vi "Demo.vi"() -> ()   [LabVIEW 2021]
uses:
  Z:/Samples/Examples/WindowsDesktop/bin/Debug/UnderAutomation.UniversalRobots.dll
  WindowsDesktop/bin/Debug/UnderAutomation.UniversalRobots.dll
panel:
  in  "Connect 2":bool
  in  "Program to load":string
  in  "Power on 6":bool
  in  "Power on 5":bool
  in  "Power on 4":bool
  in  "Power on 3":bool
  in  "Power on 2":bool
  in  "Send script":bool
  in  "Script":string
  in  "Connect":bool
  in  "IP":string
  in  "Power on":bool
  out "Z":dbl
  out "Y":dbl
  out "X":dbl
  # "Robot TCP position :"
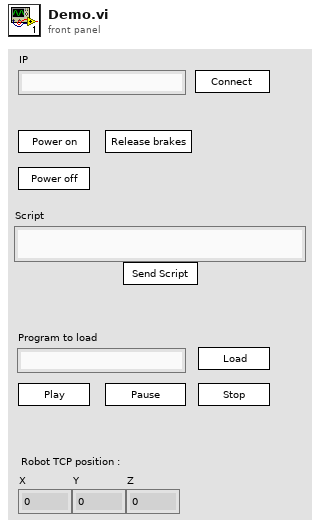
[diagram p1: front panel]
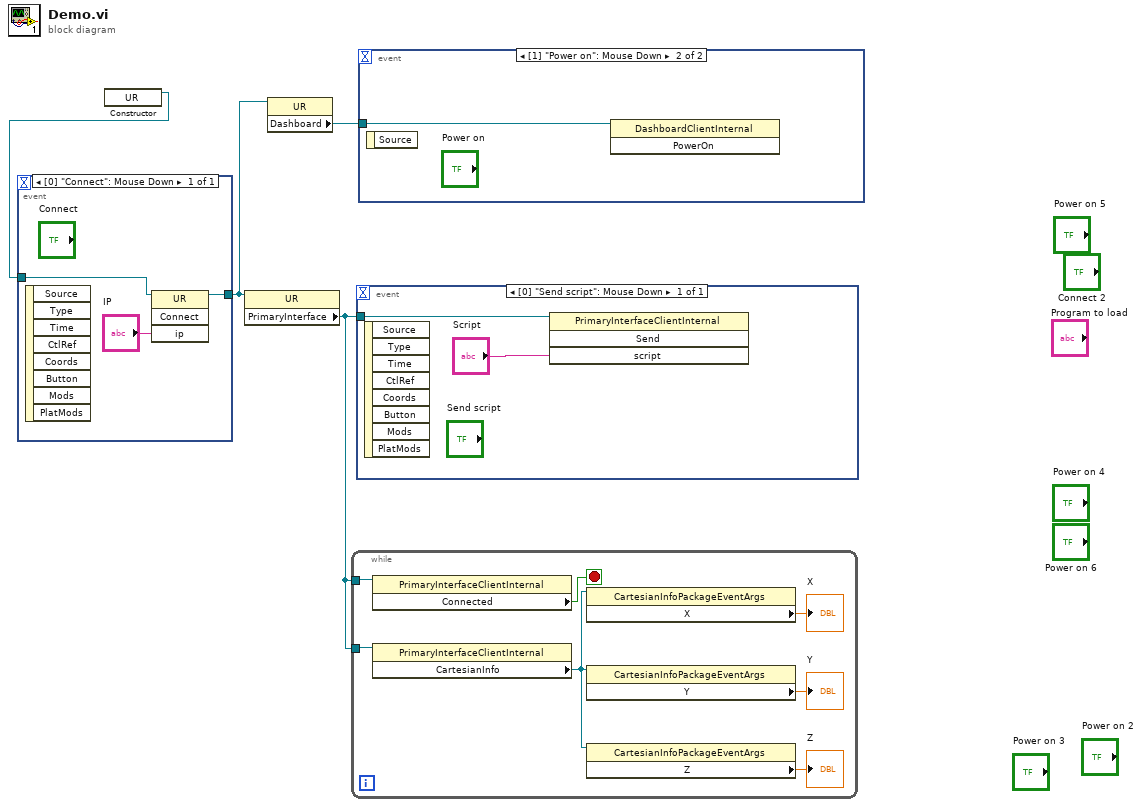
[diagram p0: block diagram]
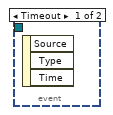
[diagram p2: hidden frame]
diagram:
  n1 = constructor class="UR"() -> (reference out=w4:refnum<k24>)  [unwired: 3 in, 2 out]
  n2 = event shown="[0] \"Connect\": Mouse Down" {
    selector: _ -> [_]
    dyn-events: _ -> [_]
    timeout: _ -> [_]
    tunnel: w4 -> [w6]
    tunnel: [w5] -> w3
    event "Connect": Mouse Down {
      n3 = event-data() -> ()  [unwired: 1 in, 8 out]
      n4 = invoke class="UR" method="Connect"(reference=w6, "ip"="IP") -> (reference out=w5:refnum<k24>)  [unwired: 2 in, 3 out]
    }
  }
  n5 = property class="UR"(reference=w3) -> ("PrimaryInterface"=w1:refnum<k24>)  [unwired: 1 in, 2 out]
  n6 = property class="UR"(reference=w3) -> ("Dashboard"=w2:refnum<k24>)  [unwired: 1 in, 2 out]
  n7 = while {
    tunnel: w1 -> [w14]
    tunnel: w1 -> [w9]
    stop <- w8 stop-if-true
    n8 = property class="PrimaryInterfaceClientInternal"(reference=w9) -> ("Connected"=w8:bool)  [unwired: 1 in, 2 out]
    n9 = property class="PrimaryInterfaceClientInternal"(reference=w14) -> ("CartesianInfo"=w13:refnum<k24>)  [unwired: 1 in, 2 out]
    n10 = property class="CartesianInfoPackageEventArgs"(reference=w13) -> ("X"=→"X":dbl)  [unwired: 1 in, 2 out]
    n11 = property class="CartesianInfoPackageEventArgs"(reference=w13) -> ("Y"=→"Y":dbl)  [unwired: 1 in, 2 out]
    n12 = property class="CartesianInfoPackageEventArgs"(reference=w13) -> ("Z"=→"Z":dbl)  [unwired: 1 in, 2 out]
  }
  n13 = event shown="[0] \"Send script\": Mouse Down" {
    selector: _ -> [_]
    dyn-events: _ -> [_]
    timeout: _ -> [_]
    tunnel: w1 -> [w16]
    event "Send script": Mouse Down {
      n14 = event-data() -> ()  [unwired: 1 in, 8 out]
      n15 = invoke class="PrimaryInterfaceClientInternal" method="Send"(reference=w16, "script"="Script") -> ()  [unwired: 2 in, 4 out]
    }
  }
  n16 = event shown="[1] \"Power on\": Mouse Down" {
    selector: _ -> [_ _]
    dyn-events: _ -> [_ _]
    timeout: _ -> [_ _]
    tunnel: w2 -> [_ w17]
    event Timeout {
      n17 = event-data() -> ()  [unwired: 1 in, 3 out]
    }
    event "Power on": Mouse Down {
      n18 = event-data() -> ()  [unwired: 1 in, 1 out]
      n19 = invoke class="DashboardClientInternal" method="PowerOn"(reference=w17) -> ()  [unwired: 2 in, 3 out]
    }
  }
